vi "HEX string to number array.vi"() -> ()   [LabVIEW 2020]
panel:
  out "Array":u8[](array[numeric]) format="%x"
  in  "String":string
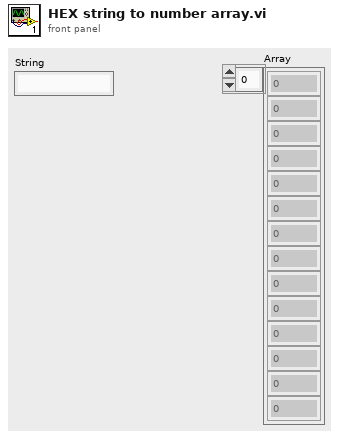
[diagram p1: front panel]
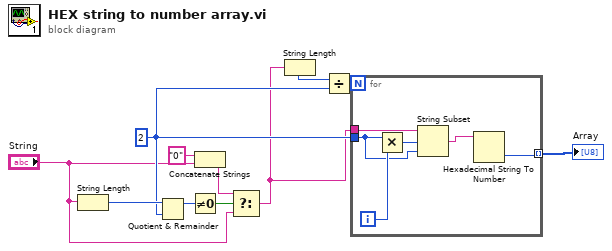
[diagram p0: block diagram]
diagram:
  w8 = 2 ("y")
  n1 = String Length(string="String") -> (length=w9:i32)
  n2 = Quotient & Remainder(x=w9, y=w8) -> (x-y*floor(x/y)=w7:i32)  [unwired: 1 out]
  n3 = Not Equal To 0?(x=w7) -> (x != 0?=w6:bool)
  n4 = Concatenate Strings("0" ("string"), "String") -> (w4:string)
  n5 = Select(t=w4, s=w6, f="String") -> (s? t:f=w2:string)
  n6 = String Length(string=w2) -> (length=w1:i32)
  n7 = Divide(x=w1, y=w8) -> (x/y=w11:dbl)
  n8 = for {
    N: w11 -> [_]
    tunnel: w2 -> [w17]
    tunnel: w8 -> [w14]
    tunnel: [w12] -> w10 mode=indexing
    i -> [w15]
    n9 = Multiply(x=w14, y=w15) -> (x*y=w16:i32)
    n10 = String Subset(string=w17, offset (0)=w16, length (rest)=w14) -> (substring=w13:string)
    n11 = Hexadecimal String To Number(string=w13) -> (number=w12:u32)  [unwired: 2 in, 1 out]
  }
  "Array" <- w10
